vi "Calculate Distance.vi"(1 "Dlong2":dbl, 2 "Dlat2":dbl, 3 "Dlong1":dbl, 4 "Dlat1":dbl) -> (0 "Distance (ft)":dbl)   [LabVIEW 2011]
uses:
  <vilib>/express/express arith-compare/Formula/XNode/ExpressFormulaBlockNode.xnode
panel:
  out "CurLatRad":dbl
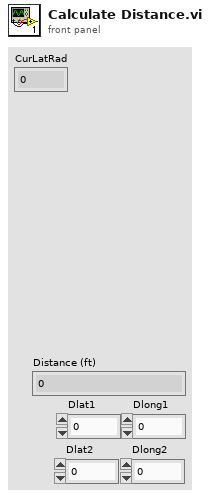
[diagram p1: front panel]
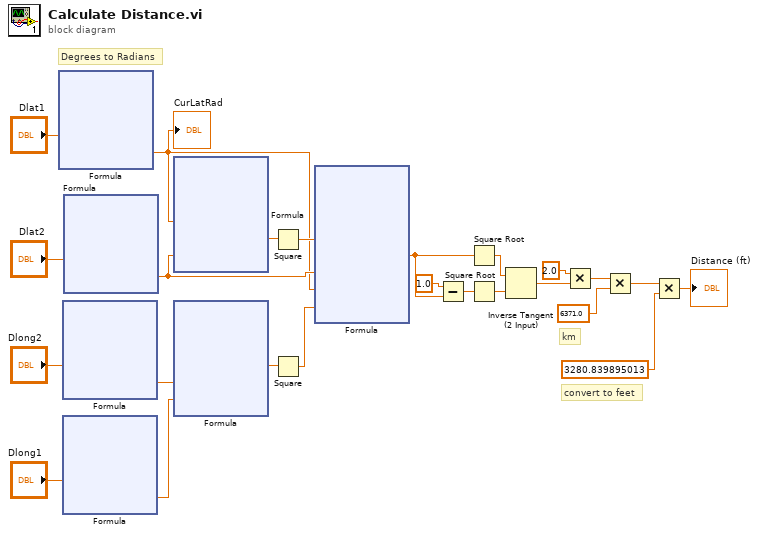
[diagram p0: block diagram]
diagram:
  # "convert to feet"
  # "km"
  # "Degrees to Radians"
  n1 = xnode "Formula"("Dlat1"="Dlat1") -> ("Result"=w17:dbl)  [unwired: 1 in, 1 out]
  "CurLatRad" <- w17
  n2 = xnode "Formula"("Dlong2"="Dlong2") -> ("Result"=w23:dbl)  [unwired: 1 in, 1 out]
  n3 = xnode "Formula"("Dlong1"="Dlong1") -> ("Result"=w22:dbl)  [unwired: 1 in, 1 out]
  n4 = xnode "Formula"("Dlat2"="Dlat2") -> ("Result"=w18:dbl)  [unwired: 1 in, 1 out]
  n5 = xnode "Formula"("CurLatRad"=w17, "DesLatRad"=w18) -> ("Result"=w24:dbl)  [unwired: 1 in, 1 out]
  n6 = xnode "Formula"("DesLongRad"=w23, "CurLongRad"=w22) -> ("Result"=w21:dbl)  [unwired: 1 in, 1 out]
  n7 = Square(x=w24) -> (x^2=w19:dbl)
  n8 = Square(x=w21) -> (x^2=w20:dbl)
  n9 = xnode "Formula"("Part1"=w19, "DesLatRad"=w18, "CurLatRad"=w17, "Part2"=w20) -> ("Result"=w15:dbl)  [unwired: 1 in, 1 out]
  n10 = Subtract(x=1.0, y=w15) -> (x-y=w13:dbl)
  n11 = Square Root(x=w15) -> (sqrt(x)=w14:dbl)
  n12 = Square Root(x=w13) -> (sqrt(x)=w7:dbl)
  n13 = Inverse Tangent (2 Input)(1:w7, 2:w14) -> (0:w12:dbl)
  n14 = Multiply(x=2.0, y=w12) -> (x*y=w10:dbl)
  n15 = Multiply(x=w10, y=6371.0) -> (x*y=w8:dbl)
  n16 = Multiply(x=w8, y=3280.839895013) -> (x*y=→"Distance (ft)":dbl)
